vi "6.feladat.vi"() -> ()   [LabVIEW 2015]
uses:
  <vilib>/Analysis/5stat.llb/RMS (DBL).vi
  <vilib>/Analysis/NI_AALPro.lvlib
panel:
  out "tri_array":dbl[](array[numeric])
  out "tri_Ueff":dbl
  out "háromszög jel":dynamicdata(graph)
  out "saw_array":dbl[](array[numeric])
  out "st_Ueff":dbl
  out "fûrész jel":dynamicdata(graph)
  out "sq_Ueff":dbl
  out "sq_array":dbl[](array[numeric])
  out "négyszög jel 2":dynamicdata(graph)
  in  "Frekvencia":dbl
  out "sin_Ueff":dbl
  out "sin_array":dbl[](array[numeric])
  out "Szinuszos jel":dynamicdata(graph)
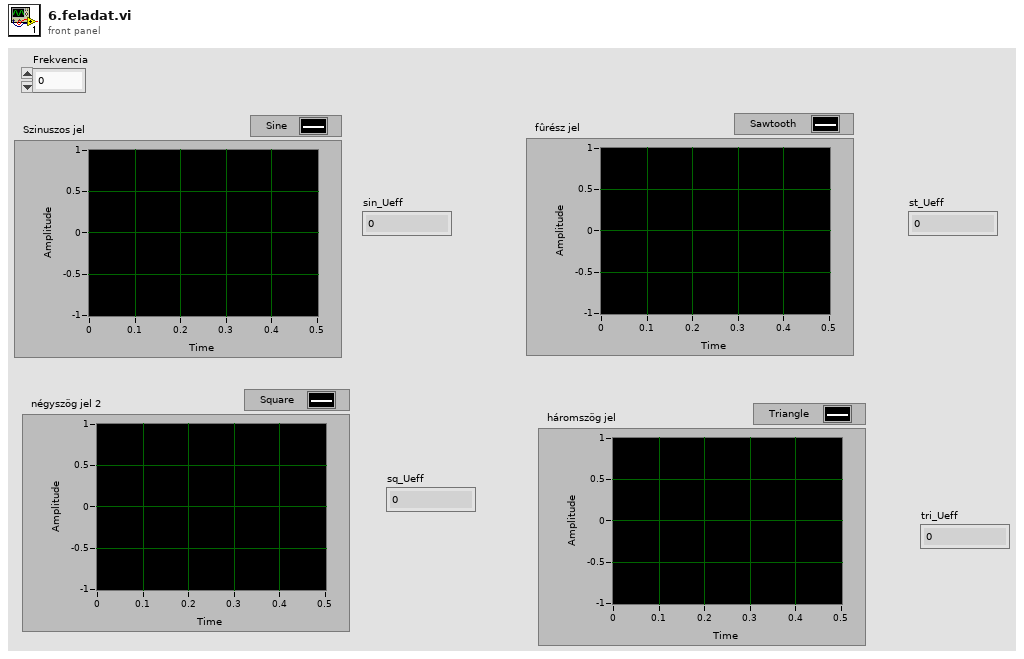
[diagram p1: front panel]
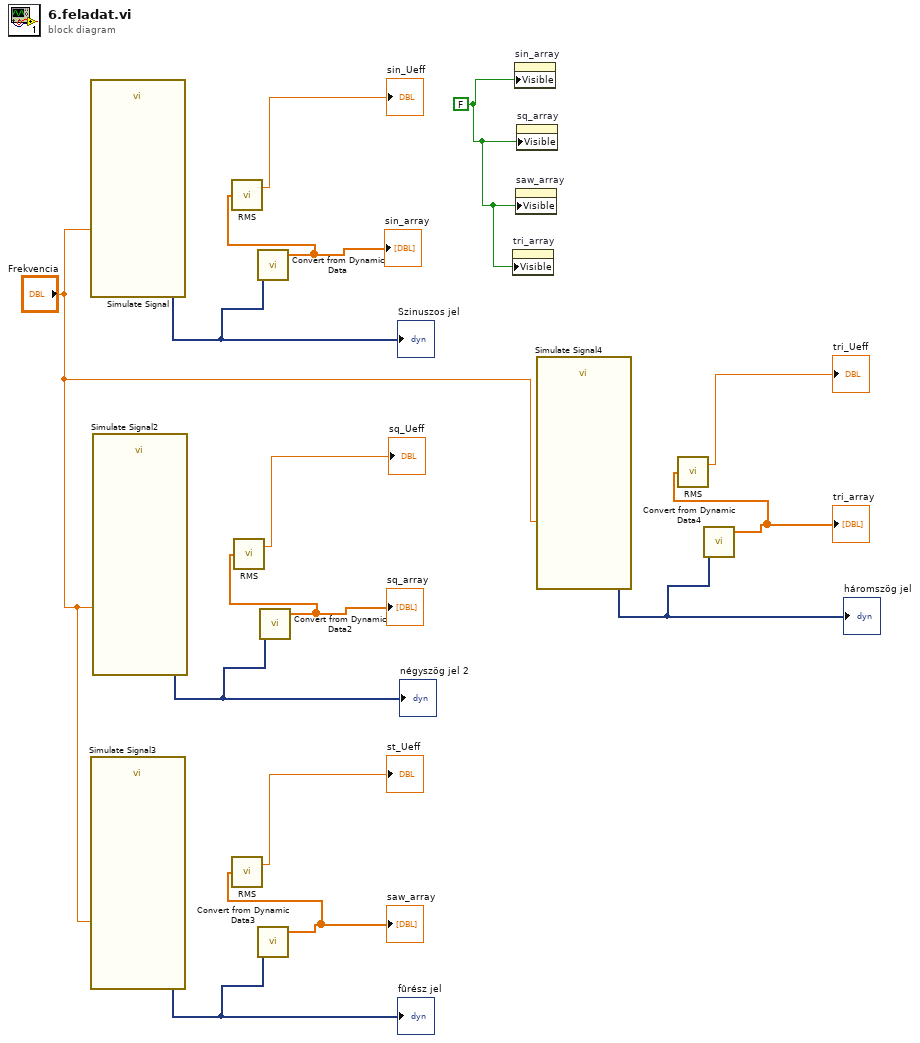
[diagram p0: block diagram]
diagram:
  w1 = FALSE
  n1 = call "Simulate Signal"("Frequency"="Frekvencia") -> ("Sine"=w14:dynamicdata)  [unwired: 13 in, 1 out]
  "Szinuszos jel" <- w14
  n2 = call "Simulate Signal3"("Frequency"="Frekvencia") -> ("Sawtooth"=w8:dynamicdata)  [unwired: 13 in, 1 out]
  "fûrész jel" <- w8
  n3 = call "Simulate Signal2"("Frequency"="Frekvencia") -> ("Square"=w11:dynamicdata)  [unwired: 13 in, 1 out]
  "négyszög jel 2" <- w11
  n4 = call "Convert from Dynamic Data"("Dynamic Data Type"=w14) -> ("Array"=w13:dbl[])  [unwired: 3 in]
  "sin_array" <- w13
  n5 = call-poly <vilib>:"RMS.vi"("X"=w13) -> ("rms value"=→"sin_Ueff":dbl)  [unwired: 1 out]
  n6 = call "Convert from Dynamic Data3"("Dynamic Data Type"=w8) -> ("Array"=w6:dbl[])  [unwired: 3 in]
  "saw_array" <- w6
  n7 = call-poly <vilib>:"RMS.vi"("X"=w6) -> ("rms value"=→"st_Ueff":dbl)  [unwired: 1 out]
  n8 = call "Convert from Dynamic Data2"("Dynamic Data Type"=w11) -> ("Array"=w10:dbl[])  [unwired: 3 in]
  "sq_array" <- w10
  n9 = call-poly <vilib>:"RMS.vi"("X"=w10) -> ("rms value"=→"sq_Ueff":dbl)  [unwired: 1 out]
  n10 = property on="tri_array" class="Arr (strict)"("Visible"=w1) -> ()  [unwired: 2 in, 2 out]
  n11 = property on="sin_array" class="Arr (strict)"("Visible"=w1) -> ()  [unwired: 2 in, 2 out]
  n12 = property on="saw_array" class="Arr (strict)"("Visible"=w1) -> ()  [unwired: 2 in, 2 out]
  n13 = property on="sq_array" class="Arr (strict)"("Visible"=w1) -> ()  [unwired: 2 in, 2 out]
  n14 = call "Simulate Signal4"("Frequency"="Frekvencia") -> ("Triangle"=w5:dynamicdata)  [unwired: 13 in, 1 out]
  "háromszög jel" <- w5
  n15 = call "Convert from Dynamic Data4"("Dynamic Data Type"=w5) -> ("Array"=w3:dbl[])  [unwired: 3 in]
  "tri_array" <- w3
  n16 = call-poly <vilib>:"RMS.vi"("X"=w3) -> ("rms value"=→"tri_Ueff":dbl)  [unwired: 1 out]
